vi "Chamber_Status_Moitor7.vi"() -> ()   [LabVIEW 2019]
uses:
  <vilib>/DAQmx/read.llb/DAQmx Read (Analog DBL 1Chan 1Samp).vi
  <vilib>/DAQmx/create/channels.llb/DAQmx Create Channel (AI-Temperature-Thermocouple).vi
  <vilib>/Instr/_visa.llb/VISA Configure Serial Port (Instr).vi
  <vilib>/Utility/file.llb/Write Delimited Spreadsheet (string).vi
  <vilib>/DAQmx/miscellaneous.llb/DAQmx Fill In Error Info.vi
panel:
  out "Setpoint [sccm]":dbl format="%_3p"
  in  "Desired Pressure [Torr]":dbl format="%.2e"
  in  "Control":bool
  in  "Email reminder":bool=TRUE
  in  "Pressure, KJLC (COM4)":refnum<visa-resource-name>="COM4"
  in  "LN2 temp, CVi (Dev4/ai0)":tag="Dev4/ai0"
  in  "He temp, LS211 (COM5)":refnum<visa-resource-name>="COM5"
  in  "MFC":bool
  in  "Setpoint (max 300)":dbl
  out "Pressure [psia]":dbl format="%.2f"
  out "Temperature [K]":dbl format="%.2f"
  out "Mass Flow [sccm]":dbl format="%.2f"
  out "Setpoint [sccm]":dbl format="%_3f"
  out "Gas":string
  in  "MFC, Alicat (COM6)":refnum<visa-resource-name>="COM6"
  in  "Record interval [s]":u32=10
  out "Status Check":string
  out "Gas":string
  out "Cryo pump":string
  in  "Cryo pump":bool
  out "Roots pump":string
  in  "Roots pump":bool
  out "Total":string[][](array[string])
  out "Mechanical pump":string
  in  "Mechanical pump":bool
  in  "File Title":string="Plasma test"
  out "Current":timestamp format="%<%m/%d/%y %I:%M:%S %p>T"
  out "Start":timestamp format="%<%m/%d/%y %I:%M:%S %p>T"
  out "Total":string
  out "He Temp":dbl format="%.2g"
  out "He Temp [C]":dbl format="%.2g"
  out "error at VISA Read":errorcluster {"code" format="%.0x"}
  out "LN2 Temp [C]":dbl format="%.2g"
  out "LN2 Temp":dbl format="%.2f"
  out "error at LS211 Config":errorcluster {"code" format="%.0x"}
  out "error at LS211 Read":errorcluster {"code" format="%.0x"}
  out "Waveform Chart":waveform(dbl)[](graph)
  out "Pressure":dbl format="%.2e"
  in  "stop":bool
  # "Chamber Status"
  # "MFC Status"
  # "Feedback Control"
  # "[Torr]"
  # "Operating System"
  # "[K]"
  # "System"
  # "Lap"
  # "[C]"
  # "[K]"
  # "[C]"
  # "Timer"
  # "Port/Channel"
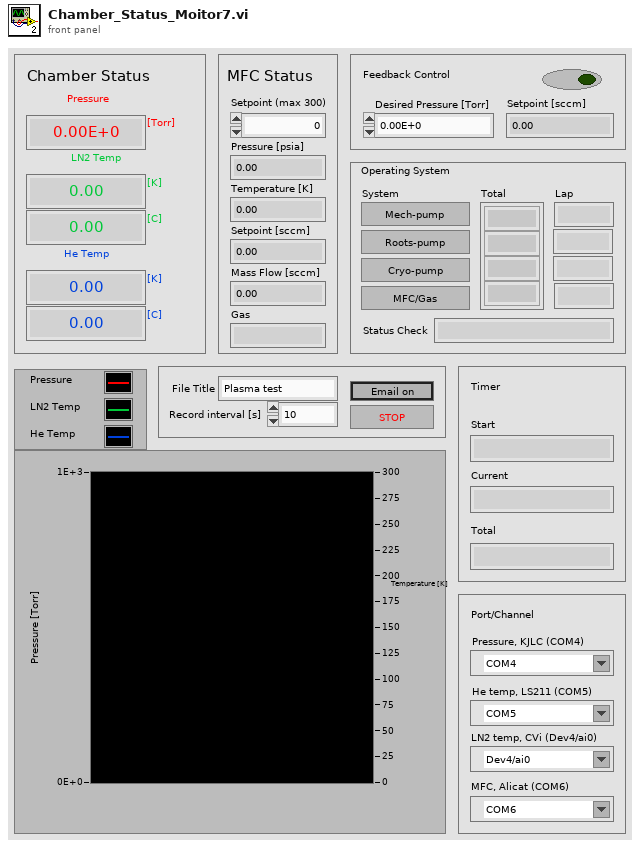
[diagram p1: front panel]
types:
  T1 = enum8{"2400", "9600", "19200", "38400", "57600", "115200", "Unknown"}
  T2 = cluster{"Unit ID":string, "Baud Rate":enum8{"2400", "9600", "19200", "38400", "57600", "115200", "Unknown"}, "MFC, Alicat (COM6)":refnum<visa-resource-name>}
  T3 = cluster{"Absolute Pressure":bool, "Gauge/Diff. Pressure":bool, "Barometric Pressure":bool, "Temperature":bool, "Volumetric":bool, "Mass":bool, "Setpoint":bool, "Valve Drive":bool, "Totalizer":bool, "Totalizer Timer":bool, "Totalizer Average Flow":bool, "Totalizer Peak Flow":bool, "Gas Selected":bool, "Tot. Timer Format":u16}
  T4 = cluster{"Controller Full Scale":dbl, "Controller Select":u16, "Control Range":enum16{"Normal", "Inverted", "Bidirectional", "Unknown"}}
  T5 = cluster{"Absolute Pressure":dbl, "Gauge/Diff. Pressure":dbl, "Barometric Pressure":dbl, "Temperature":dbl, "Volumetric Flow":dbl, "Mass Flow":dbl, "Setpoint":dbl, "Valve Drive":dbl, "Totalizer":dbl, "[hr]":dbl, "[min]":dbl, "[sec]":dbl, "Totalizer Average Flow":dbl, "Totalizer Peak Flow":dbl, "Gas selected":string}
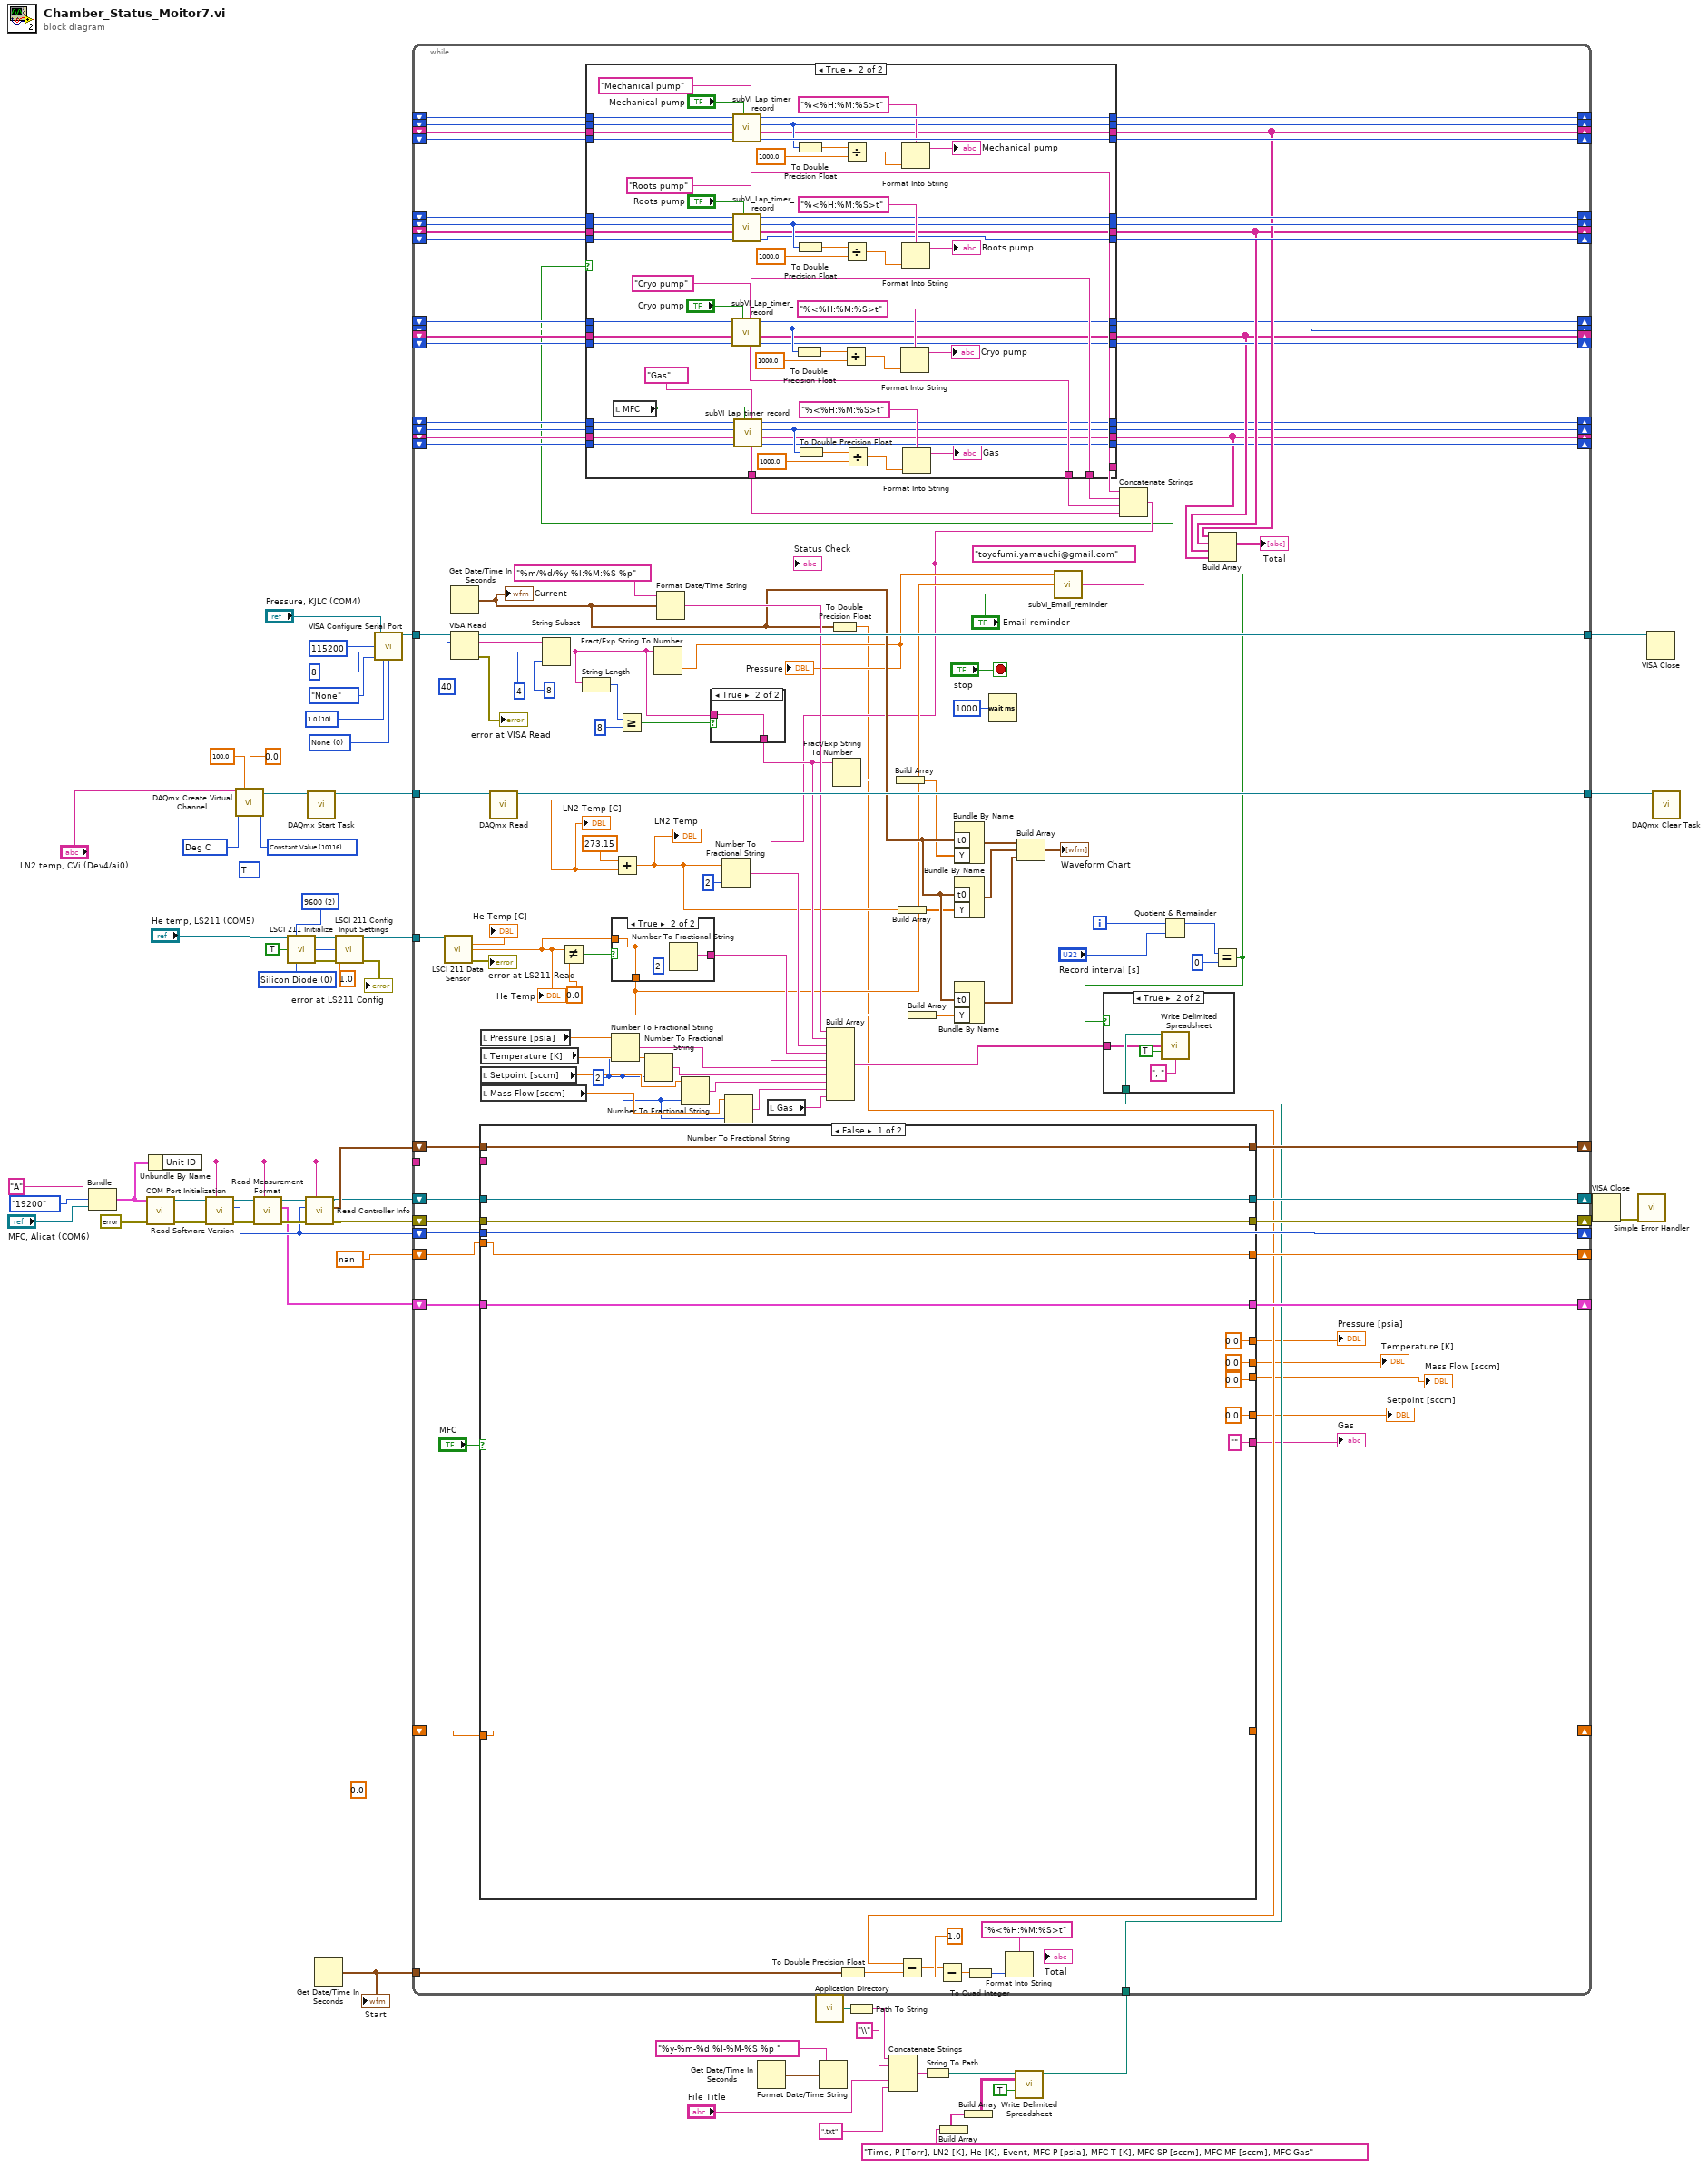
[diagram p0: block diagram]
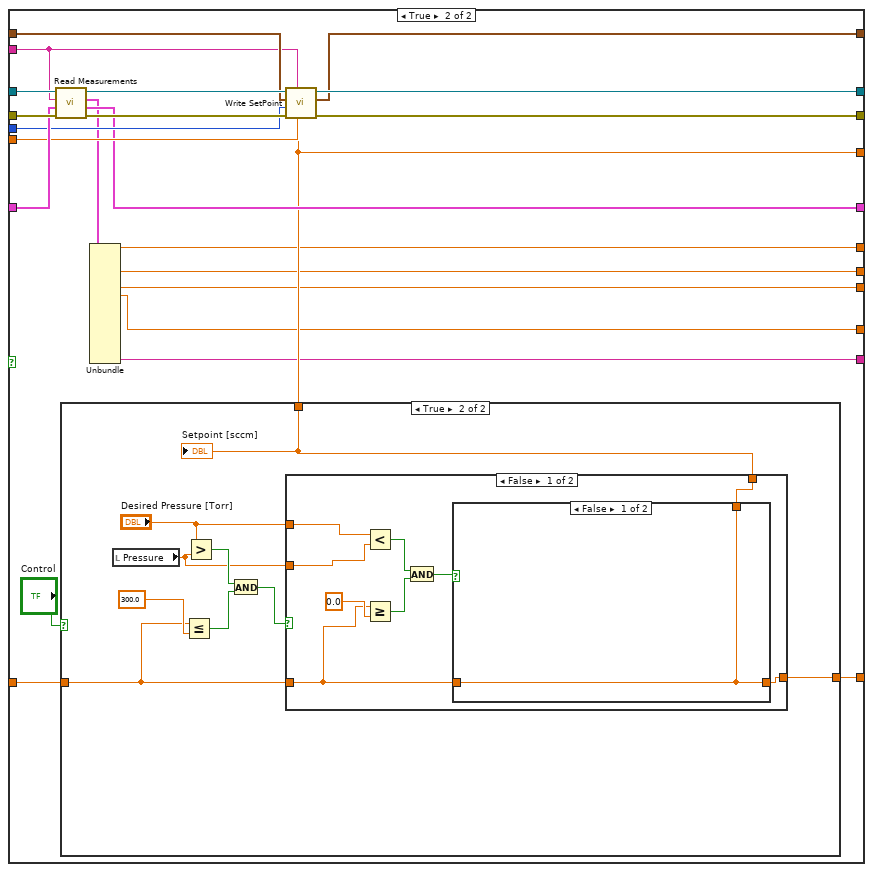
[diagram p2: hidden frame]
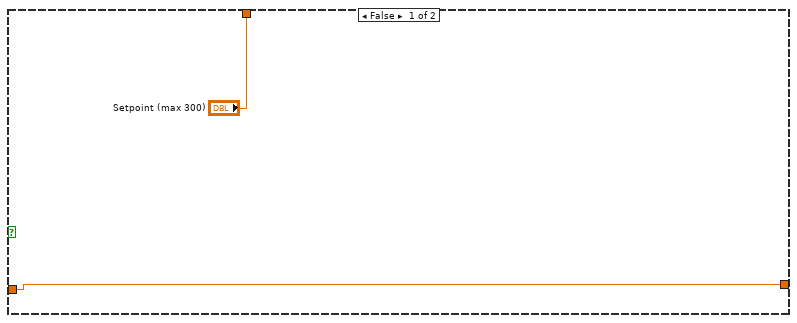
[diagram p3: hidden frame]
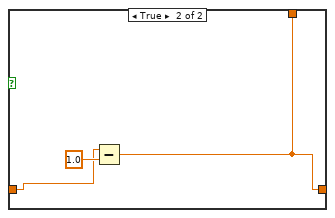
[diagram p4: hidden frame]
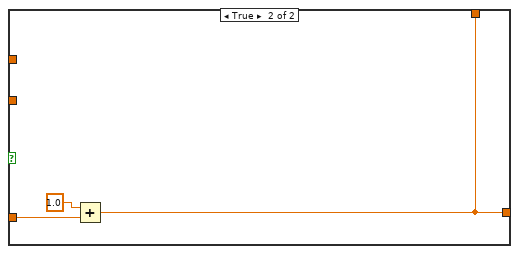
[diagram p5: hidden frame]
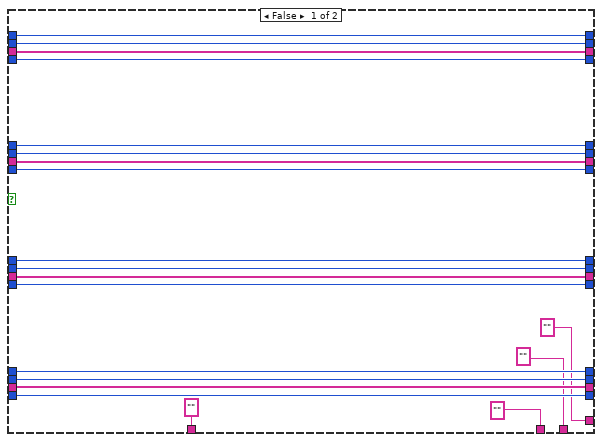
[diagram p6: hidden frame]
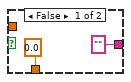
[diagram p8: hidden frame]
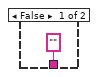
[diagram p9: hidden frame]
diagram:
  w43 = 10086 items=["J"=10072, "K"=10073, "N"=10077, "R"=10082, "S"=10085, "T"=10086, "B"=10047, "E"=10055] ("thermocouple type")
  w44 = 10116 items=["Built-In"=10200, "Constant Value"=10116, "Channel"=10113] ("cjc source")
  w45 = 10143 items=["Deg C"=10143, "Deg F"=10144, "Kelvins"=10325, "Deg R"=10145, "From Custom Scale"=10065] ("units")
  w62 = i8 0 items=["Silicon Diode", "GaAIAS Diode", "100 Ohm Platinum/250", "100 Ohm Platinum/500", "1000 Ohm Platinum", "NTC RTD"] ("Sensor Type (0: Silicon Diode)")
  w63 = 2 items=["300", "1200", "9600"] ("Baud Rate [2: 9600]")
  w50 = u16 0 items=["None", "XON/XOFF", "RTS/CTS", "XON/XOFF & RTS/CTS", "DTR/DSR", "XON/XOFF & DTR/DSR"] ("flow control (0:none)")
  w51 = u16 10 items=["1.0"=10, "1.5"=15, "2.0"=20] ("stop bits (10: 1 bit)")
  n1 = Bundle("Unit ID"="A", "Baud Rate"=T1."19200", "MFC, Alicat (COM6)"="MFC, Alicat (COM6)") -> (w12:T2)  [unwired: 1 in]
  n2 = call "COM Port Initialization.vi"("error in (no error)"=errorcluster {"status"=FALSE, "code"=0, "source"=""}, "Communication Settings"=w12) -> ("error out"=w18:errorcluster, "VISA Session Out"=w19:refnum<visa-resource-name>)  [unwired: 8 in]
  n3 = Unbundle By Name(w12) -> ("Unit ID"=w10:string)
  n4 = call "Read Software Version.vi"("Unit ID (A)"=w10, "error in"=w18, "VISA Session In"=w19) -> ("error out"=w17:errorcluster, "Software Version"=w9:u8, "VISA Session Out"=w16:refnum<visa-resource-name>)  [unwired: 6 in]
  n5 = call-poly <vilib>:"DAQmx Create Virtual Channel.vi"("maximum value"=100.0, "minimum value"=0.0, "physical channels"="LN2 temp, CVi (Dev4/ai0)", "cjc source"=w44, "units"=w45, "thermocouple type"=w43) -> ("task out"=w40:refnum<k21>)  [unwired: 8 in, 1 out]
  n6 = call "Read Measurement Format.vi"("Unit ID (A)"=w10, "error in"=w17, "VISA Session In"=w16) -> ("error out"=w21:errorcluster, "Data Frame Format"=w7:T3, "VISA Session Out"=w20:refnum<visa-resource-name>)  [unwired: 6 in]
  n7 = call "LSCI 211 Initialize.vi"("Instr. Descriptor (ASRL1::INSTR)"="He temp, LS211 (COM5)", "Reset (T: Reset)"=TRUE, "Baud Rate [2: 9600]"=w63) -> ("VISA session"=w60:refnum<visa-resource-name>, "error out"=w49:errorcluster)  [unwired: 11 in]
  n8 = call "Read Controller Info.vi"("Unit ID (A)"=w10, "error in"=w21, "Software Version"=w9, "VISA Session In"=w20) -> ("error out"=w6:errorcluster, "Controller Info out"=w11:T4, "VISA Session Out"=w5:refnum<visa-resource-name>)  [unwired: 4 in, 1 out]
  n9 = call <vilib>:"DAQmx Start Task.vi"("task/channels in"=w40) -> ("task out"=w42:refnum<k21>)  [unwired: 13 in, 1 out]
  n10 = Get Date/Time In Seconds() -> (seconds since 1Jan1904=w39:timestamp)
  "Start" <- w39
  n11 = call "LSCI 211 Config Input Settings.vi"("VISA session"=w60, "Sensor Type (0: Silicon Diode)"=w62, "Curve Number (0)"=1.0, "error in (no error)"=w49) -> ("dup VISA session"=w58:refnum<visa-resource-name>, "error out"=→"error at LS211 Config":errorcluster)  [unwired: 10 in]
  n12 = call-poly "VISA Configure Serial Port"("VISA resource name"="Pressure, KJLC (COM4)", "baud rate (9600)"=u32 115200, "data bits (8)"=8 ("offset"), "parity (0:none)"=enum16{"None", "Odd", "Even", "Mark", "Space"}."None", "stop bits (10: 1 bit)"=w51, "flow control (0:none)"=w50) -> ("VISA resource name out"=w56:refnum<visa-resource-name>)  [unwired: 8 in, 1 out]
  n13 = Get Date/Time In Seconds() -> (seconds since 1Jan1904=w35:timestamp)
  n14 = call <vilib>:"Application Directory.vi"() -> ("Application Directory"=w36:path)
  n15 = Format Date/Time String(time format string (%c)="%y-%m-%d %I-%M-%S %p ", seconds (now)=w35) -> (date/time string=w26:string)  [unwired: 1 in]
  n16 = Path To String(path=w36) -> (string=w37:string)
  n17 = Concatenate Strings(w37, "\\" ("string"), w26, "File Title", ".txt" ("string")) -> (w38:string)
  n18 = String To Path(string=w38) -> (path=w32:path)
  n19 = Build Array("Time, P [Torr], LN2 [K], He [K], Event, MFC P [psia], MFC T [K], MFC SP [sccm], MFC MF [sccm], MFC Gas") -> (w29:string[])
  n20 = Build Array(w29) -> (w28:string[][])
  n21 = call-poly <vilib>:"Write Delimited Spreadsheet.vi"("file path (dialog if empty)"=w32, "2D data"=w28, "append to file? (new file:F)"=TRUE) -> ("new file path (Not A Path if cancelled)"=w31:path)  [unwired: 11 in, 1 out]
  n22 = while {
    tunnel: [w186] -> w64
    tunnel: w56 -> [w149]
    tunnel: w58 -> [w182]
    tunnel: w42 -> [w171]
    tunnel: [w170] -> w41
    tunnel: w39 -> [w168]
    tunnel: w31 -> [w72]
    shift-right: [w137] -> _
    shift-left: _ -> [w136]
    shift-right: [w131] -> _
    shift-left: _ -> [w135]
    shift-right: [w120] -> _
    shift-left: _ -> [w134]
    shift-right: [w133] -> _
    shift-left: _ -> [w132]
    shift-right: [w130] -> _
    shift-left: _ -> [w129]
    shift-right: [w128] -> _
    shift-left: _ -> [w127]
    shift-right: [w119] -> _
    shift-left: _ -> [w126]
    shift-right: [w125] -> _
    shift-left: _ -> [w124]
    shift-right: [w118] -> _
    shift-left: _ -> [w115]
    shift-right: [w117] -> _
    shift-left: _ -> [w114]
    shift-right: [w111] -> _
    shift-left: _ -> [w113]
    shift-right: [w116] -> _
    shift-left: _ -> [w112]
    shift-right: [w108] -> _
    shift-left: _ -> [w104]
    shift-right: [w105] -> _
    shift-left: _ -> [w102]
    shift-right: [w107] -> _
    shift-left: _ -> [w103]
    shift-right: [w106] -> _
    shift-left: _ -> [w101]
    tunnel: w10 -> [w90]
    shift-right: [w89] -> _
    shift-left: w11 -> [w91]
    shift-right: [w88] -> w4
    shift-left: w5 -> [w92]
    shift-right: [w87] -> _
    shift-left: w9 -> [w87]
    shift-right: [w86] -> _
    shift-left: nan ("Setpoint") -> [w94]
    shift-right: [w85] -> _
    shift-left: w7 -> [w95]
    shift-right: [w84] -> w3
    shift-left: w6 -> [w93]
    shift-right: [w71] -> _
    shift-left: 0.0 ("Setpoint (max 300) 2") -> [w70]
    i -> [w140]
    stop <- "stop" stop-if-true
    w74 = i16 2 ("precision (6)")
    n23 = call "LSCI 211 Data Sensor.vi"("VISA session"=w182) -> ("Celsius Reading"=→"He Temp [C]":dbl, "Kelvin Reading"=w150:dbl, "error out"=→"error at LS211 Read":errorcluster)  [unwired: 9 in, 3 out]
    "He Temp" <- w150
    n24 = Get Date/Time In Seconds() -> (seconds since 1Jan1904=w157:timestamp)
    "Current" <- w157
    n25 = VISA Read(VISA resource name=w149, byte count=u32 40) -> (VISA resource name out=w186:refnum<visa-resource-name>, read buffer=w188:string, error out=→"error at VISA Read":errorcluster)  [unwired: 1 in, 1 out]
    n26 = case shown="False" "MFC" {
      tunnel: w93 -> [w200 w225]
      tunnel: w92 -> [w201 w224]
      tunnel: w95 -> [w198 w223]
      tunnel: [w201 w221] -> w88
      tunnel: w91 -> [w202 w220]
      tunnel: [w202 w219] -> w89
      tunnel: w94 -> [w199 w218]
      tunnel: w90 -> [_ w217]
      tunnel: [w200 w215] -> w84
      tunnel: [w199 w211] -> w86
      tunnel: w87 -> [_ w214]
      tunnel: [w198 w213] -> w85
      tunnel: [w197 w210] -> w71
      tunnel: w70 -> [w197 w209]
      tunnel: ["" ("Gas selected") w207] -> w69
      tunnel: [0.0 ("Setpoint") w206] -> w68
      tunnel: [0.0 ("Mass Flow") w205] -> w67
      tunnel: [0.0 ("Temperature") w204] -> w66
      tunnel: [0.0 ("Absolute Pressure") w203] -> w65
      frame False {
      }
      frame True {
        n27 = call "Read Measurements.vi"("error in"=w225, "Data Frame Format In"=w223, "Unit ID (A)"=w217, "VISA Session In"=w224) -> ("error out"=w216:errorcluster, "Data Frame Format Out"=w213:T3, "Data Cluster"=w208:T5, "VISA Session Out"=w222:refnum<visa-resource-name>)  [unwired: 4 out]
        n28 = case shown="True" "Control" {
          tunnel: ["Setpoint (max 300)" w230] -> w211
          tunnel: [w226 w233] -> w210
          tunnel: w209 -> [w226 w228]
          frame False {
          }
          frame True {
            n29 = local read "Pressure"() -> (w231:dbl)
            n30 = Less Or Equal?(x=w228, y=300.0 ("Setpoint (max 300) 2")) -> (x <= y?=w235:bool)
            n31 = Greater?(x="Desired Pressure [Torr]", y=w231) -> (0:w236:bool)
            n32 = And(x=w236, y=w235) -> (x .and. y?=w234:bool)
            n33 = case shown="False" w234 {
              tunnel: [w244 w251] -> w230
              tunnel: [w245 w251] -> w233
              tunnel: w228 -> [w237 w250]
              tunnel: "Desired Pressure [Torr]" -> [w243 _]
              tunnel: w231 -> [w239 _]
              frame False {
                n34 = Less?(x=w243, y=w239) -> (x < y?=w241:bool)
                n35 = Greater Or Equal?(x=w237, y=0.0 ("x")) -> (x >= y?=w240:bool)
                n36 = And(x=w241, y=w240) -> (x .and. y?=w242:bool)
                n37 = case shown="False" w242 {
                  tunnel: w237 -> [w246 w248]
                  tunnel: [w246 w247] -> w245
                  tunnel: [w246 w247] -> w244
                  frame False {
                  }
                  frame True {
                    n38 = Subtract(x=w248, y=1.0) -> (x-y=w247:dbl)
                  }
                }
              }
              frame True {
                n39 = Add(x=1.0, y=w250) -> (x+y=w251:dbl)
              }
            }
            "Setpoint [sccm]" <- w230
          }
        }
        n40 = Unbundle(w208) -> ("Absolute Pressure"=w203:dbl, "Temperature"=w204:dbl, "Mass Flow"=w205:dbl, "Setpoint"=w206:dbl, "Gas selected"=w207:string)  [unwired: 10 out]
        n41 = call "Write SetPoint.vi"("Setpoint"=w211, "Previous Setpoint"=w218, "Unit ID (A)"=w217, "error in"=w216, "Software Version"=w214, "Controller Info out"=w220, "VISA Session In"=w222) -> ("error out"=w215:errorcluster, "Controller Info out"=w219:T4, "VISA Session Out"=w221:refnum<visa-resource-name>)  [unwired: 1 in, 1 out]
      }
    }
    "Pressure [psia]" <- w65
    "Temperature [K]" <- w66
    "Mass Flow [sccm]" <- w67
    "Setpoint [sccm]" <- w68
    "Gas" <- w69
    n42 = local read "Pressure [psia]"() -> (w82:dbl)
    n43 = local read "Temperature [K]"() -> (w79:dbl)
    n44 = local read "Setpoint [sccm]"() -> (w78:dbl)
    n45 = local read "Mass Flow [sccm]"() -> (w75:dbl)
    n46 = call-poly <vilib>:"DAQmx Read.vi"("task/channels in"=w171) -> ("task out"=w170:refnum<k21>, "data"=w169:dbl)  [unwired: 12 in, 1 out]
    "LN2 Temp [C]" <- w169
    n47 = String Subset(string=w188, offset (0)=4, length (rest)=8 ("length (rest)")) -> (substring=w151:string)
    n48 = Not Equal?(x=w150, y=0.0) -> (x != y?=w174:bool)
    n49 = String Length(string=w151) -> (length=w183:i32)
    n50 = case shown="True" w174 {
      tunnel: w150 -> [_ w343]
      tunnel: ["" w345] -> w167
      tunnel: [0.0 ("Kelvin Reading") w343] -> w138
      frame False {
      }
      frame True {
        n51 = Number To Fractional String(number=w343, precision (6)=i16 2) -> (F-format string=w345:string)  [unwired: 2 in]
      }
    }
    n52 = Number To Fractional String(number=w82, precision (6)=w74) -> (F-format string=w81:string)  [unwired: 2 in]
    n53 = Add(x=273.15 ("y"), y=w169) -> (x+y=w153:dbl)
    "LN2 Temp" <- w153
    n54 = Greater Or Equal?(x=w183, y=8 ("x")) -> (x >= y?=w184:bool)
    n55 = Number To Fractional String(number=w79, precision (6)=w74) -> (F-format string=w80:string)  [unwired: 2 in]
    n56 = Fract/Exp String To Number(string=w151) -> (number=w143:dbl)  [unwired: 3 in, 1 out]
    "Pressure" <- w143
    n57 = Format Date/Time String(time format string (%c)="%m/%d/%y %I:%M:%S %p" ("format string"), seconds (now)=w157) -> (date/time string=w165:string)  [unwired: 1 in]
    n58 = Number To Fractional String(number=w78, precision (6)=w74) -> (F-format string=w77:string)  [unwired: 2 in]
    n59 = case shown="True" w184 {
      tunnel: w151 -> [_ w347]
      tunnel: ["" ("read buffer") w347] -> w161
      frame False {
      }
      frame True {
      }
    }
    n60 = Number To Fractional String(number=w153, precision (6)=i16 2) -> (F-format string=w163:string)  [unwired: 2 in]
    n61 = Number To Fractional String(number=w75, precision (6)=w74) -> (F-format string=w76:string)  [unwired: 2 in]
    n62 = local read "Gas"() -> (w83:string)
    n63 = To Double Precision Float(number=w157) -> (double precision float=w73:dbl)
    n64 = Fract/Exp String To Number(string=w161) -> (number=w155:dbl)  [unwired: 3 in, 1 out]
    n65 = To Double Precision Float(number=w168) -> (double precision float=w172:dbl)
    n66 = Build Array(w155) -> (w154:dbl[])
    n67 = Build Array(w153) -> (w152:dbl[])
    n68 = Subtract(x=w73, y=w172) -> (x-y=w147:dbl)
    n69 = Build Array(w138) -> (w156:dbl[])
    n70 = Subtract(x=w147, y=1.0) -> (x-y=w146:dbl)
    n71 = Bundle By Name("t0"=w157, "Y"=w154) -> (w160:waveform(dbl))  [unwired: 1 in]
    n72 = Bundle By Name("t0"=w157, "Y"=w152) -> (w159:waveform(dbl))  [unwired: 1 in]
    n73 = Bundle By Name("t0"=w157, "Y"=w156) -> (w158:waveform(dbl))  [unwired: 1 in]
    n74 = To Quad Integer(1:w146) -> (0:w177:i64)
    n75 = Wait (ms)(milliseconds to wait=u32 1000) -> ()  [unwired: 1 out]
    n76 = Format Into String(format string="%<%H:%M:%S>t", w177) -> (resulting string=→"Total":string)  [unwired: 2 in, 1 out]
    n77 = Build Array(w160, w159, w158) -> (→"Waveform Chart":waveform(dbl)[])
    n78 = call "subVI_Email_reminder.vi"("Receipt email address"="toyofumi.yamauchi@gmail.com", "Email reminder"="Email reminder", "He temp"=w138, "Pressure"=w143) -> ()
    n79 = Quotient & Remainder(x=w140, y="Record interval [s]") -> (x-y*floor(x/y)=w141:u32)  [unwired: 1 out]
    n80 = Equal?(x=w141, y=u32 0) -> (x = y?=w98:bool)
    n81 = case shown="True" w98 {
      tunnel: [w272 w336] -> w137
      tunnel: w136 -> [w272 w335]
      tunnel: w135 -> [w271 w332]
      tunnel: w134 -> [w270 w331]
      tunnel: [w269 w330] -> w133
      tunnel: w132 -> [w269 w329]
      tunnel: [w271 w323] -> w131
      tunnel: [w268 w316] -> w130
      tunnel: w129 -> [w268 w315]
      tunnel: [w267 w314] -> w128
      tunnel: w127 -> [w267 w313]
      tunnel: w126 -> [w266 w312]
      tunnel: [w265 w311] -> w125
      tunnel: w124 -> [w265 w310]
      tunnel: ["" ("Notes") w309] -> w122
      tunnel: ["" ("Notes") w308] -> w121
      tunnel: [w270 w307] -> w120
      tunnel: [w266 w306] -> w119
      tunnel: [w264 w297] -> w118
      tunnel: [w263 w296] -> w117
      tunnel: [w261 w295] -> w116
      tunnel: w115 -> [w264 w294]
      tunnel: w114 -> [w263 w293]
      tunnel: w113 -> [w262 w292]
      tunnel: w112 -> [w261 w291]
      tunnel: [w262 w290] -> w111
      tunnel: ["" ("Notes") w289] -> w110
      tunnel: ["" ("Notes") w282] -> w109
      tunnel: [w260 w281] -> w108
      tunnel: [w259 w280] -> w107
      tunnel: [w257 w279] -> w106
      tunnel: [w258 w278] -> w105
      tunnel: w104 -> [w260 w277]
      tunnel: w103 -> [w259 w276]
      tunnel: w102 -> [w258 w275]
      tunnel: w101 -> [w257 w274]
      frame False {
      }
      frame True {
        n82 = local read "MFC"() -> (w273:bool)
        n83 = call "subVI_Lap_timer_record.vi"("Name"="Cryo pump", "Boolean"="Cryo pump", "1/0 in"=w291, "Lapped time in"=w292, "Lap time in"=w293, "Total time in"=w294) -> ("1/0 out"=w295:i32, "Lapped time out"=w290:string[], "Lap time out"=w296:u32, "Total time out"=w297:u32, "Notes"=w289:string)  [unwired: 1 in]
        n84 = call "subVI_Lap_timer_record.vi"("Name"="Mechanical pump", "Boolean"="Mechanical pump", "1/0 in"=w329, "Lapped time in"=w331, "Lap time in"=w332, "Total time in"=w335) -> ("1/0 out"=w330:i32, "Lapped time out"=w307:string[], "Lap time out"=w323:u32, "Total time out"=w336:u32, "Notes"=w309:string)  [unwired: 1 in]
        n85 = call "subVI_Lap_timer_record.vi"("Name"="Roots pump", "Boolean"="Roots pump", "1/0 in"=w310, "Lapped time in"=w312, "Lap time in"=w313, "Total time in"=w315) -> ("1/0 out"=w311:i32, "Lapped time out"=w306:string[], "Lap time out"=w314:u32, "Total time out"=w316:u32, "Notes"=w308:string)  [unwired: 1 in]
        n86 = call "subVI_Lap_timer_record.vi"("Name"="Gas", "Boolean"=w273, "1/0 in"=w274, "Lapped time in"=w275, "Lap time in"=w276, "Total time in"=w277) -> ("1/0 out"=w279:i32, "Lapped time out"=w278:string[], "Lap time out"=w280:u32, "Total time out"=w281:u32, "Notes"=w282:string)  [unwired: 1 in]
        n87 = To Double Precision Float(number=w296) -> (double precision float=w303:dbl)
        n88 = To Double Precision Float(number=w323) -> (double precision float=w328:dbl)
        n89 = To Double Precision Float(number=w314) -> (double precision float=w320:dbl)
        n90 = To Double Precision Float(number=w280) -> (double precision float=w287:dbl)
        n91 = Divide(x=w303, y=1000.0 ("Factor to seconds")) -> (x/y=w300:dbl)
        n92 = Divide(x=w328, y=1000.0 ("Factor to seconds")) -> (x/y=w325:dbl)
        n93 = Divide(x=w320, y=1000.0 ("Factor to seconds")) -> (x/y=w321:dbl)
        n94 = Divide(x=w287, y=1000.0 ("Factor to seconds")) -> (x/y=w284:dbl)
        n95 = Format Into String(format string="%<%H:%M:%S>t", w300) -> (resulting string=→"Cryo pump":string)  [unwired: 2 in, 1 out]
        n96 = Format Into String(format string="%<%H:%M:%S>t", w325) -> (resulting string=→"Mechanical pump":string)  [unwired: 2 in, 1 out]
        n97 = Format Into String(format string="%<%H:%M:%S>t", w321) -> (resulting string=→"Roots pump":string)  [unwired: 2 in, 1 out]
        n98 = Format Into String(format string="%<%H:%M:%S>t", w284) -> (resulting string=→"Gas":string)  [unwired: 2 in, 1 out]
      }
    }
    n99 = Concatenate Strings(w122, w121, w110, w109) -> (w99:string)
    "Status Check" <- w99
    n100 = Build Array(w165, w161, w163, w167, w99, w81, w80, w77, w76, w83) -> (w164:string[])
    n101 = case shown="True" w98 {
      tunnel: w72 -> [_ w339]
      tunnel: w164 -> [_ w337]
      frame False {
      }
      frame True {
        n102 = call-poly <vilib>:"Write Delimited Spreadsheet.vi"("file path (dialog if empty)"=w339, "1D data"=w337, "append to file? (new file:F)"=TRUE, "delimiter (\\t)"=", " ("delimiter (\\t)")) -> ()  [unwired: 10 in, 2 out]
      }
    }
    n103 = Build Array(w120, w119, w111, w105) -> (→"Total":string[][])
  }
  n104 = VISA Close(VISA resource name=w4, error in (no error)=w3) -> (error out=w2:errorcluster)
  n105 = call <vilib>:"Simple Error Handler.vi"("error in (no error)"=w2) -> ()  [unwired: 4 in, 5 out]
  n106 = VISA Close(VISA resource name=w64) -> ()  [unwired: 1 in, 1 out]
  n107 = call <vilib>:"DAQmx Clear Task.vi"("task in"=w41) -> ()  [unwired: 14 in, 1 out]
